vi "Read VISA resource name.vi"(8 "error in (no error)":errorcluster, 11 "Bobcat 640 in":refnum<class "Bobcat 640.lvclass">) -> (0 "error out":errorcluster, 2 "IMAQdx Session":T1, 3 "Bobcat 640 out":refnum<class "Bobcat 640.lvclass">)   [LabVIEW 2018, in "Bobcat 640.lvlib" / "Bobcat 640.lvclass"]
uses:
  Bobcat 640.lvclass
  <vilib>/userdefined/High Color/IMAQdx.ctl
  Bobcat 640.lvclass/Bobcat 640.ctl
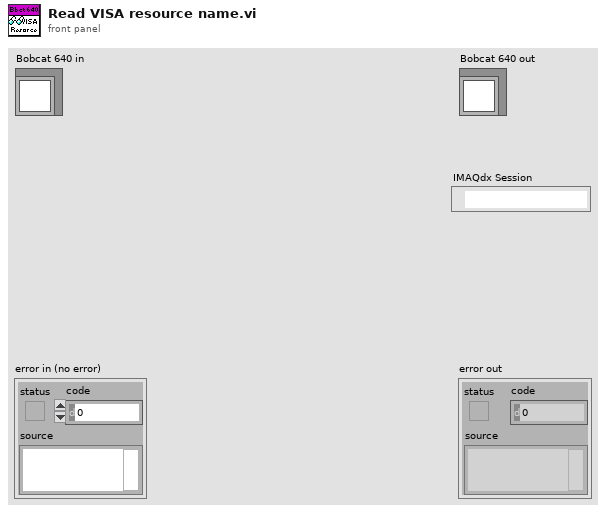
[diagram p1: front panel]
types:
  T1 = typedef "IMAQdx.ctl" = refnum<k21>
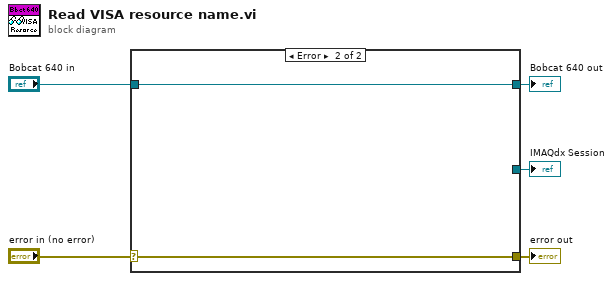
[diagram p0: block diagram]
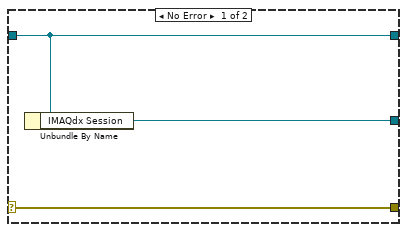
[diagram p2: hidden frame]
diagram:
  n1 = case shown="Error" "error in (no error)" {
    selector: "error in (no error)" -> [w8 w9]
    tunnel: [w8 w9] -> w4
    tunnel: [w7 w10] -> w2
    tunnel: "Bobcat 640 in" -> [w7 w10]
    tunnel: [w6 _] -> w1
    frame No Error {
      n2 = Unbundle By Name(w7) -> ("IMAQdx Session"=w6:T1)
    }
    frame Error {
    }
  }
  "error out" <- w4
  "Bobcat 640 out" <- w2
  "IMAQdx Session" <- w1
